vi "Запись в файл (SubVI).vi"(7 "Резервное сохр.":bool, 8 "error in":errorcluster, 10 "Строка параметров мишеней для сохранения":string) -> (0 "error out":errorcluster, 3 "путь к файлу ref":refnum<file>, 5 "Путь к файлу":path)   [LabVIEW 2013]
doc: "Сохранение текущей конфигурации в файл Настройки.txt, расположенный в каталоге с исполняемым файлом"
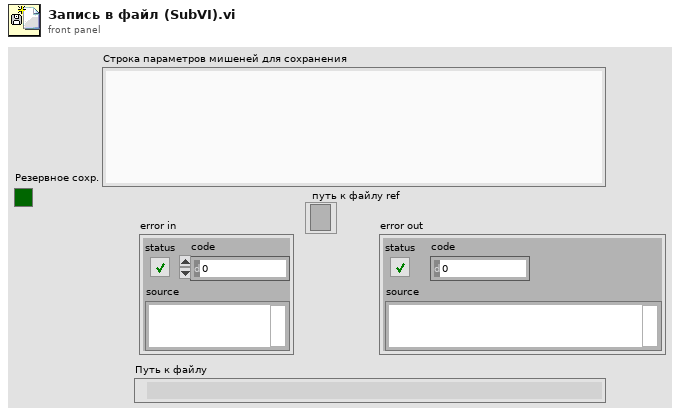
[diagram p1: front panel]
types:
  T1 = enum16{"open", "replace", "create", "open or create", "replace or create", "replace or create with confirmation"}
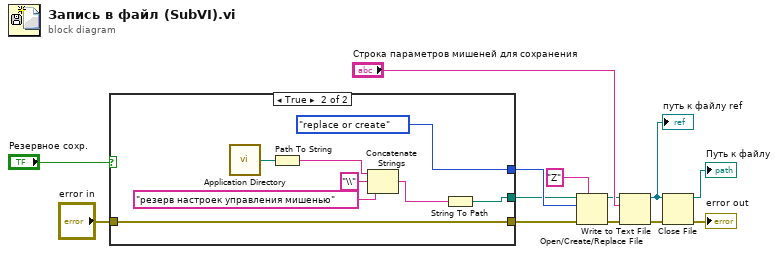
[diagram p0: block diagram]
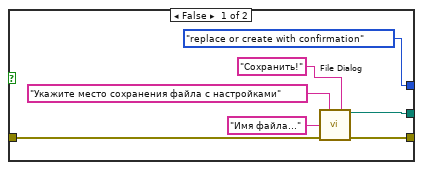
[diagram p2: hidden frame]
diagram:
  n1 = case shown="True" "Резервное сохр." {
    tunnel: [T1."replace or create with confirmation" ("operation (0:open)") T1."replace or create" ("operation (0:open)")] -> w9
    tunnel: [w19 w27] -> w6
    tunnel: [w15 w22] -> w5
    tunnel: "error in" -> [w14 w27]
    frame False {
      n2 = call "File Dialog"("prompt"="Укажите место сохранения файла с настройками" ("string"), "button label"="Сохранить!" ("string"), "default name"="Имя файла..." ("string"), "error in"=w14) -> ("selected path"=w15:path, "error out"=w19:errorcluster)  [unwired: 8 in, 2 out]
    }
    frame True {
      n3 = call <vilib>:"Application Directory.vi"() -> ("Application Directory"=w26:path)
      n4 = Path To String(path=w26) -> (string=w23:string)
      n5 = Concatenate Strings(w23, "\\" ("string"), "резерв настроек управления мишенью" ("string")) -> (w21:string)
      n6 = String To Path(string=w21) -> (path=w22:path)
    }
  }
  n7 = Open/Create/Replace File(file path (use dialog)=w5, error in=w6, prompt="Z", operation (0:open)=w9) -> (refnum out=w10:refnum<file>, error out=w8:errorcluster)  [unwired: 3 out]
  n8 = Write to Text File(file (use dialog)=w10, text="Строка параметров мишеней для сохранения", error in=w8) -> (refnum out=w12:refnum<file>, error out=w11:errorcluster)  [unwired: 1 in, 1 out]
  "путь к файлу ref" <- w12
  n9 = Close File(refnum=w12, error in=w11) -> (path=→"Путь к файлу":path, error out=→"error out":errorcluster)
